vi "Create Events.vi"(0 "Display State In":T2, 9 "Container State":T3, 11 "error in (no error)":errorcluster) -> (4 "Display State Out":T2, 8 "Events":T1, 15 "error out":errorcluster)   [LabVIEW 2015, in "TTLController.xctl"]
uses:
  TTLController.xctl
  <vilib>/_xctls/Container State.ctl
  State.ctl
  Device Classes/Base Class/TTLControlledDevice.lvclass
  Events.ctl
  Event Type.ctl
  Height Change.vi
  Event Data.ctl
  <vilib>/_xctls/XControlSupport.lvlib
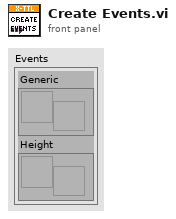
[diagram p1: front panel]
types:
  T1 = typedef "TTLController.xctl/Events.ctl" = cluster{"Generic":refnum<user-event>, "Height":refnum<user-event>}
  T2 = typedef "TTLController.xctl/State.ctl" = cluster{"Active":bool, "Device":refnum<class "TTLControlledDevice.lvclass">, "Events":T1, "Height":i32}
  T3 = typedef "XControlSupport.lvlib/Container State.ctl" = cluster{"Indicator?":bool, "Run Mode?":bool, " Refnum":refnum<vi>}
  T4 = typedef "TTLController.xctl/Height Change.vi" = cluster{"New":i32, "Old":i32, "Ref":refnum<vi>}
  T5 = typedef "TTLController.xctl/Event Data.ctl" = cluster{"Type":T6, "Data":variant}
  T6 = typedef "TTLController.xctl/Event Type.ctl" = enum16{"None", "Selection", "Edit", "Insert", "Delete", "Up", "Down"}
  T7 = cluster{"Event Data":refnum<user-event>, "Event Data":refnum<user-event>}
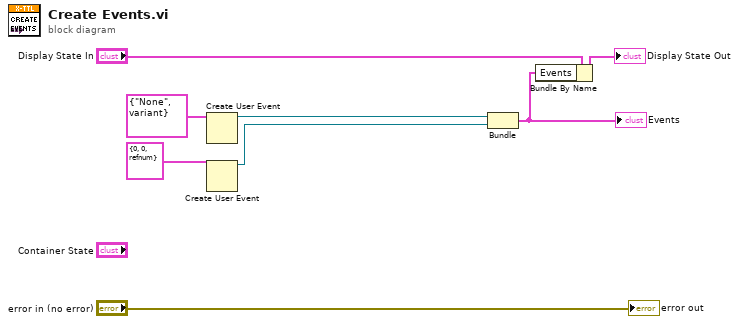
[diagram p0: block diagram]
diagram:
  n1 = Create User Event(user event datatype=T5 {"Type"=enum."None", "Data"=variant} ("Event Data")) -> (user event=w4:refnum<user-event>)  [unwired: 1 in, 1 out]
  n2 = Create User Event(user event datatype=T4 {"New"=0, "Old"=0, "Ref"=refnum} ("Event Data")) -> (user event=w1:refnum<user-event>)  [unwired: 1 in, 1 out]
  n3 = Bundle("Event Data"=w4, "Event Data"=w1) -> (w3:T7)  [unwired: 1 in]
  "Events" <- w3
  n4 = Bundle By Name(cluster="Display State In", "Events"=w3) -> (→"Display State Out":T2)
  "error out" <- "error in (no error)"
